vi "Local Transition.vi"(8 "error in (no error)":errorcluster, 9 "Target State":refnum<class "State.lvclass">, 10 "Context in":refnum<data-value>, 11 "Nested State in":refnum<class "Nested State.lvclass">) -> (0 "error out":errorcluster, 2 "Context out":refnum<data-value>, 3 "Nested State out":refnum<class "Nested State.lvclass">)   [LabVIEW 2024, in "Nested State.lvclass"]
uses:
  Nested State.lvclass
  Nested State.lvclass/Nested State.ctl
  State/State.lvclass
  Context/Context/Context.lvclass
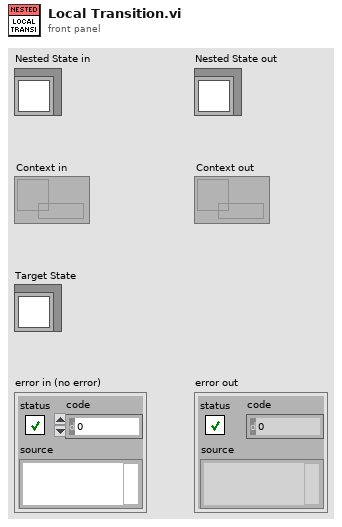
[diagram p1: front panel]
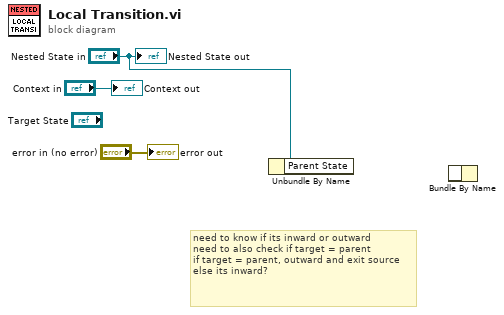
[diagram p0: block diagram]
diagram:
  # "need to know if its inward or outward\nneed to also check if target = parent\nif target = parent, outward and exit source\nelse its inward?"
  n1 = Unbundle By Name("Nested State in") -> ()  [unwired: 1 out]
  n2 = Bundle By Name() -> ()  [unwired: 2 in, 1 out]
  "error out" <- "error in (no error)"
  "Nested State out" <- "Nested State in"
  "Context out" <- "Context in"
